vi "Get Item From Index.vi"(8 "错误输入":errorcluster, 10 "Index":i32, 11 "Mlistbox Ref":refnum<vi>) -> (0 "错误输出":errorcluster, 2 "Item":string[](array[string]), 3 "Mlistbox Ref Dup":refnum<vi>)   [LabVIEW 2012, in "Mlistbox Tools.lvlib"]
uses:
  Mlistbox Tools.lvlib
  ListBox/Custom Type/Read and Write Mode.ctl
  Property/Set and Get ItemNames.vi
  ListBox/Listbox Tool.lvlib
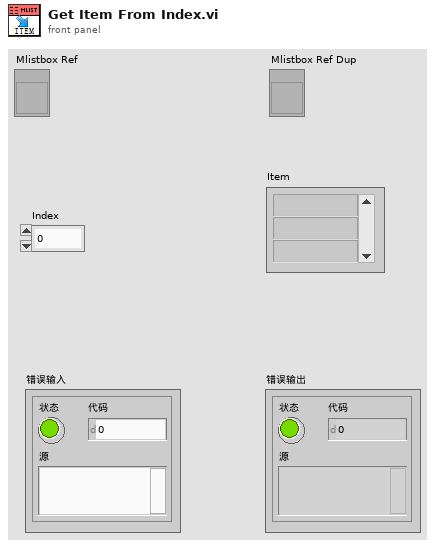
[diagram p1: front panel]
types:
  T1 = typedef "Listbox Tool.lvlib/Read and Write Mode.ctl" = enum16{"Read", "Write"}
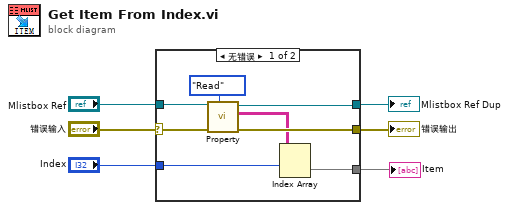
[diagram p0: block diagram]
diagram:
  n1 = case shown="无错误" "错误输入" {
    selector: "错误输入" -> [w12 w16]
    tunnel: [w10 w16] -> w5
    tunnel: "Mlistbox Ref" -> [w14 w15]
    tunnel: [w11 w15] -> w3
    tunnel: "Index" -> [w8 _]
    tunnel: [w7 _] -> w1
    frame No Error {
      n2 = call-poly "Property.vi"("Mode"=Read_and_Write_Mode."Read", "错误输入"=w12, "Mlistbox Ref"=w14) -> ("错误输出"=w10:errorcluster, "ItemNames Out"=w9:string[][], "Mlistbox Ref Dup"=w11:refnum<vi>)  [unwired: 6 in]
      n3 = Index Array(array=w9, index (row)=w8) -> (element=w7:string[])  [unwired: 1 in]
    }
    frame Error {
    }
  }
  "Mlistbox Ref Dup" <- w3
  "错误输出" <- w5
  "Item" <- w1
